vi "Round Number.vi"(11 "Square in":refnum<class "Square.lvclass">) -> (2 "Round Number":u32)   [LabVIEW 2020, in "SquareBattle.lvlib" / "Square.lvclass"]
doc: "Provides the current round number of the game. This can be used to provide time coordinated actions within a team."
uses:
  Square.lvclass
  Square.lvclass/Square.ctl
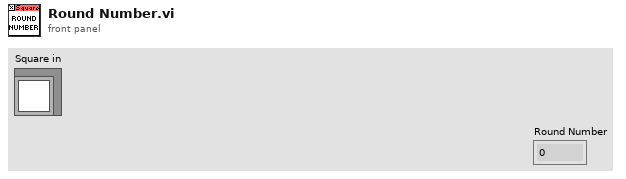
[diagram p1: front panel]
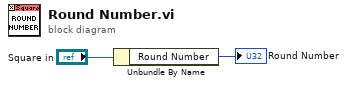
[diagram p0: block diagram]
diagram:
  n1 = Unbundle By Name("Square in") -> ("Round Number"=→"Round Number":u32)
